vi "Test.vi"() -> ()   [LabVIEW 2020]
uses:
  D:/Git/Graph-Extensions-LabVIEW-master/LV2014/Libraries/Graph Module/netDxf_2.4.2/bin/Release/netDxf.dll
  Libraries/Graph Module/netDxf_2.4.2/bin/Release/netDxf.dll
panel:
  out "error out":errorcluster
  in  "path":path=path "D:/Git/Graph-Extensions-LabVIEW-master/LV2014/dxf/163_CAD2000_.dxf"
  in  "error in (no error)":errorcluster
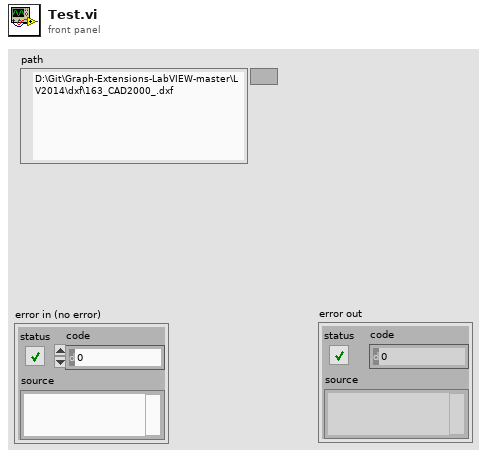
[diagram p1: front panel]
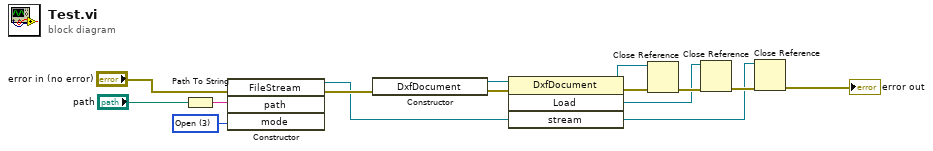
[diagram p0: block diagram]
diagram:
  w13 = 3 items=["CreateNew"=1, "Create"=2, "Open"=3, "OpenOrCreate"=4, "Truncate"=5, "Append"=6] ("mode")
  n1 = Path To String(path="path") -> (string=w12:string)
  n2 = constructor class="FileStream"(error in="error in (no error)", "path"=w12, "mode"=w13) -> (reference out=w3:refnum<k24>, error out=w9:errorcluster)  [unwired: 2 in, 3 out]
  n3 = constructor class="DxfDocument"(error in=w9) -> (reference out=w10:refnum<k24>, error out=w11:errorcluster)  [unwired: 2 in, 1 out]
  n4 = invoke class="DxfDocument" method="Load"(reference=w10, error in=w11, "stream"=w3) -> (reference out=w7:refnum<k24>, error out=w8:errorcluster, "Load"=w5:refnum<k24>)  [unwired: 1 in, 1 out]
  n5 = Close Reference(reference=w7, error in (no error)=w8) -> (error out=w6:errorcluster)
  n6 = Close Reference(reference=w5, error in (no error)=w6) -> (error out=w4:errorcluster)
  n7 = Close Reference(reference=w3, error in (no error)=w4) -> (error out=→"error out":errorcluster)
